vi "OFDM-SIM同步.vi"(0 "接收的串行数据流":cdb[](array[numeric]), 1 "信噪比":dbl) -> (2 "定时频偏":i32[](array[numeric]), 3 "频率偏移(Hz)":dbl[](array[numeric]), 4 "相位":dbl[](array[numeric]), 5 "幅度":dbl[](array[numeric]))   [LabVIEW 2018]
panel:
  out "大小 5":i32
  out "大小 4":i32
  out "大小 3":i32
  out "大小 2":i32
  out "大小":i32
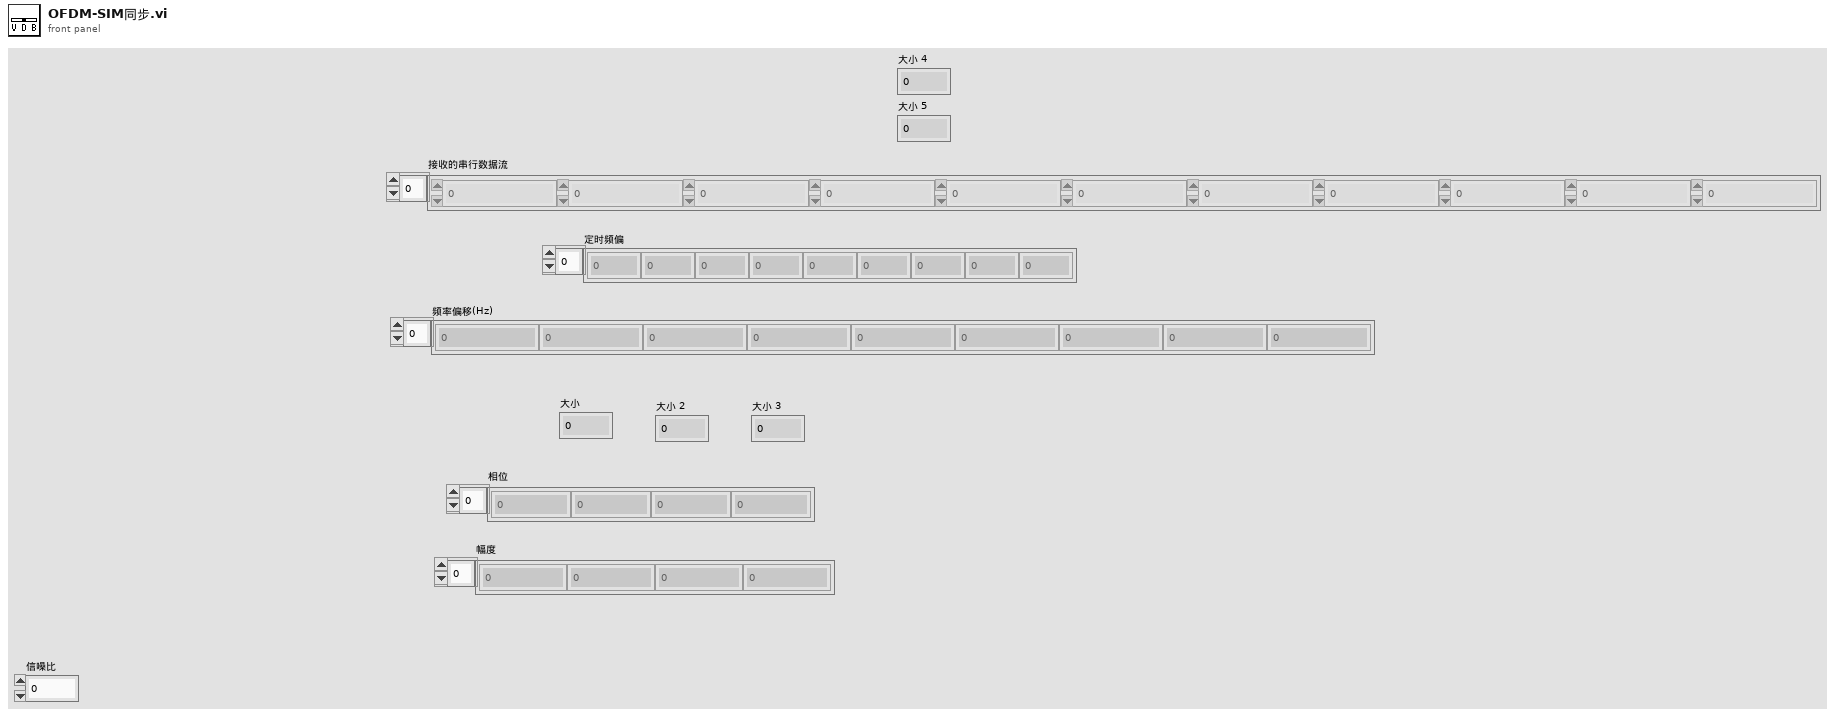
[diagram p1: front panel]
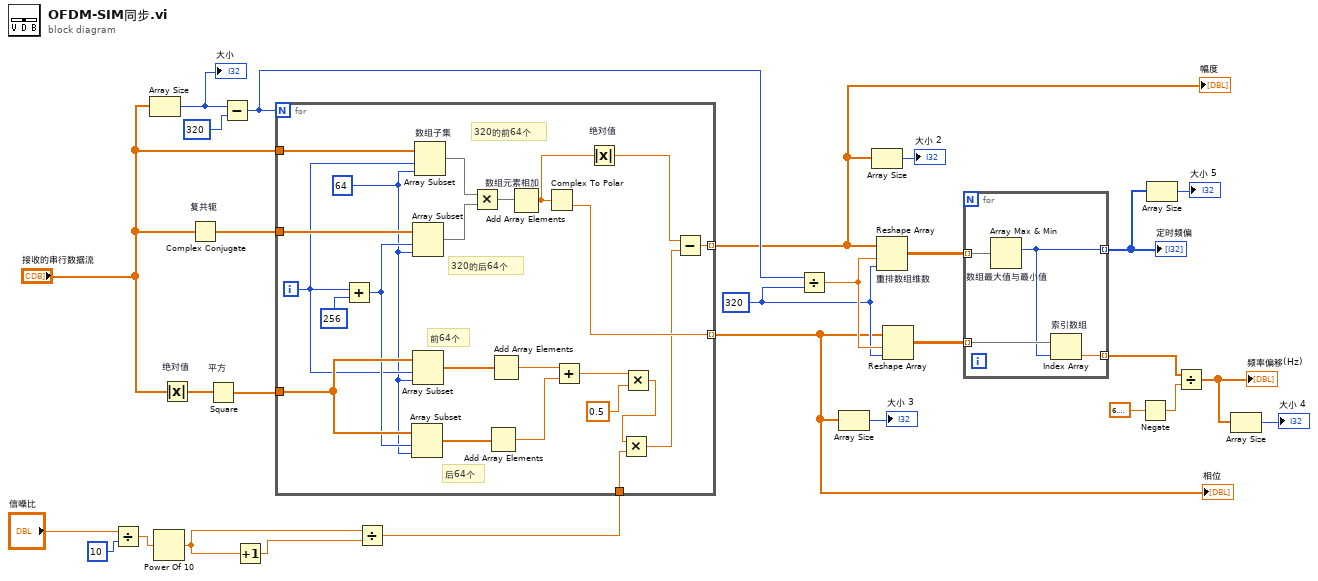
[diagram p0: block diagram]
diagram:
  w20 = 320 ("y")
  n1 = Divide(x="信噪比", y=10) -> (x/y=w4:dbl)
  n2 = Array Size(array="接收的串行数据流") -> (size(s)=w28:i32)
  "大小" <- w28
  n3 = Power Of 10(x=w4) -> (10^x=w3:dbl)
  n4 = Absolute Value "绝对值"(x="接收的串行数据流") -> (abs(x)=w26:dbl[])
  n5 = Complex Conjugate "复共轭"(1:"接收的串行数据流") -> (0:w25:cdb[])
  n6 = Square "平方"(x=w26) -> (x^2=w24:dbl[])
  n7 = Subtract(x=w28, y=320) -> (x-y=w23:i32)
  n8 = Increment(x=w3) -> (x+1=w6:dbl)
  n9 = Divide(x=w3, y=w6) -> (x/y=w1:dbl)
  n10 = for {
    N: w23 -> [_]
    tunnel: "接收的串行数据流" -> [w51]
    tunnel: w25 -> [w50]
    tunnel: w24 -> [w48]
    tunnel: [w37] -> w8 mode=indexing
    tunnel: [w36] -> w10 mode=indexing
    tunnel: w1 -> [w32]
    i -> [w46]
    w35 = 64 ("长度")
    # "前64个"
    # "后64个"
    # "320的后64个"
    # "320的前64个"
    n11 = Add(x=w46, y=256) -> (x+y=w47:i32)
    n12 = Array Subset(array=w48, index=w47, length=w35) -> (w45:dbl[])
    n13 = Array Subset(array=w50, index=w47, length=w35) -> (w42:cdb[])
    n14 = Array Subset(array=w48, index=w46, length=w35) -> (w44:dbl[])
    n15 = Array Subset "数组子集"(array=w51, index=w46, length=w35) -> (w43:cdb[])
    n16 = Multiply(x=w43, y=w42) -> (x*y=w41:cdb[])
    n17 = Add Array Elements(numeric array=w45) -> (sum=w39:dbl)
    n18 = Add Array Elements(numeric array=w44) -> (sum=w40:dbl)
    n19 = Add Array Elements "数组元素相加"(numeric array=w41) -> (sum=w31:cdb)
    n20 = Complex To Polar ("复数至极坐标转换")(r * e^(i*theta)=w31) -> (theta=w36:dbl)  [unwired: 1 out]
    n21 = Add(x=w40, y=w39) -> (x+y=w34:dbl)
    n22 = Absolute Value "绝对值"(x=w31) -> (abs(x)=w29:dbl)
    n23 = Multiply(x=w34, y=0.5) -> (x*y=w33:dbl)
    n24 = Multiply(x=w33, y=w32) -> (x*y=w30:dbl)
    n25 = Subtract(x=w29, y=w30) -> (x-y=w37:dbl)
  }
  "相位" <- w10
  "幅度" <- w8
  n26 = Divide(x=w23, y=w20) -> (x/y=w21:dbl)
  n27 = Array Size(array=w10) -> (size(s)=→"大小 3":i32)
  n28 = Array Size(array=w8) -> (size(s)=→"大小 2":i32)
  n29 = Reshape Array "重排数组维数"(w8, w21, w20) -> (w19:dbl[][])
  n30 = Reshape Array(w10, w21, w20) -> (w18:dbl[][])
  n31 = for {
    tunnel: w19 -> [w55] mode=indexing
    tunnel: w18 -> [w54] mode=indexing
    tunnel: [w53] -> w14 mode=indexing
    tunnel: [w52] -> w9 mode=indexing
    n32 = Array Max & Min "数组最大值与最小值"(array=w55) -> (max index (indices)=w53:i32)  [unwired: 3 out]
    n33 = Index Array "索引数组"(array=w54, index=w53) -> (element=w52:dbl)
  }
  "定时频偏" <- w14
  n34 = Negate(x=6.283185307179586) -> (-x=w16:dbl)
  n35 = Array Size(array=w14) -> (size(s)=→"大小 5":i32)
  n36 = Divide(x=w9, y=w16) -> (x/y=w13:dbl[])
  "频率偏移(Hz)" <- w13
  n37 = Array Size(array=w13) -> (size(s)=→"大小 4":i32)
